vi "Close UI.vi"(11 "Settings UI in":refnum<class "Settings UI.lvclass">) -> (3 "Settings UI out":refnum<class "Settings UI.lvclass">)   [LabVIEW 2020, in "Output Sequencer.lvlib" / "Settings UI.lvclass"]
uses:
  Settings UI.lvclass
  Settings UI.lvclass/Settings UI.ctl
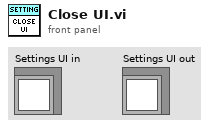
[diagram p1: front panel]
types:
  T1 = enum32{"Invalid", "Standard", "Closed", "Hidden", "Minimized", "Maximized"}
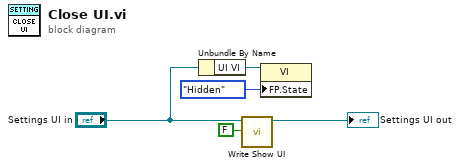
[diagram p0: block diagram]
diagram:
  n1 = Unbundle By Name("Settings UI in") -> ("UI VI"=w5:refnum<vi>)
  n2 = call "Write Show UI.vi"("Applied Settings"=FALSE, "Settings UI in"="Settings UI in") -> ("Settings UI out"=→"Settings UI out":refnum<class "Settings UI.lvclass">)  [unwired: 8 in, 1 out]
  n3 = property class="VI"(reference=w5, "FP.State"=T1."Hidden" ("Front Panel Window:State")) -> ()  [unwired: 1 in, 2 out]
